vi "Data Access.vi"(8 "error in (no error)":errorcluster, 10 "Data Access Handler":refnum<class "Data Access Handler.lvclass">, 11 "List Instrument Msg in":refnum<class "List Instruments Msg.lvclass">) -> (0 "error out":errorcluster, 3 "List Instrument Msg out":refnum<class "List Instruments Msg.lvclass">)   [LabVIEW 2020, in "Instrument Handler.lvlib" / "List Instruments Msg.lvclass"]
doc: "Expose class private data to the front panel while letting the Data Access Handler class act on the data."
uses:
  List Instruments Msg.lvclass
  C:/Current projects/WS/Framework/Framework/Actors/Instrument Handler/Instrument Handler Messages/Instrument Handler Response Msg/Instrument Handler Response Msg.lvclass
  C:/Current projects/WS/PPL/HDH.Actor Framework.Core.Msg.lvlibp/Flex Msg/Flex Msg.lvclass
  PPL/HDH.Actor Framework.Core.Msg.lvlibp/Flex Msg/Data Access Handlers/Data Access Handler/Data Access Handler.lvclass
  PPL/HDH.Actor Framework.Core.Publisher.lvlibp/Messages/Response Msg/Response Core/Controls/Ctl_SendFunction.ctl
  PPL/HDH.Actor Framework.Core.Actor.lvlibp/1abvi3w/vi.lib/ActorFramework/Message Enqueuer/Message Priority.ctl
  Instrument Handler Response Msg/Instrument Handler Response Msg.lvclass/Instrument Handler Response Msg.ctl
  Instrument Handler Response Msg/Instrument Handler Response Msg.lvclass
  PPL/HDH.Actor Framework.Core.Publisher.lvlibp
  PPL/HDH.Actor Framework.Core.Actor.lvlibp/1abvi3w/vi.lib/ActorFramework/Message Enqueuer/Message Enqueuer.lvclass
panel:
  in  "Message Priority":T1=enum."Normal"
  in  "Send Function(Await Reply)":T2=enum."Await Reply"
  in  "Timeout if Waiting(-1ms)":i32=-1
  in  "Publish Data?(T)":bool=TRUE
  in  "Cancel":bool
  in  "OK":bool
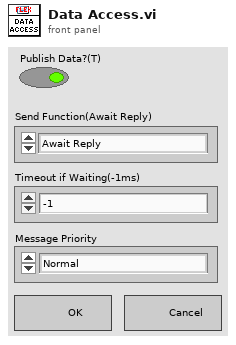
[diagram p1: front panel]
types:
  T1 = typedef "HDH.Actor Framework.Core.Actor.lvlibp/Message Enqueuer.lvclass/Message Priority.ctl" = enum16{"Low", "Normal", "High"}
  T2 = typedef "HDH.Actor Framework.Core.Publisher.lvlibp/Ctl_SendFunction.ctl" = enum16{"Send and Forget", "Request Reply", "Await Reply"}
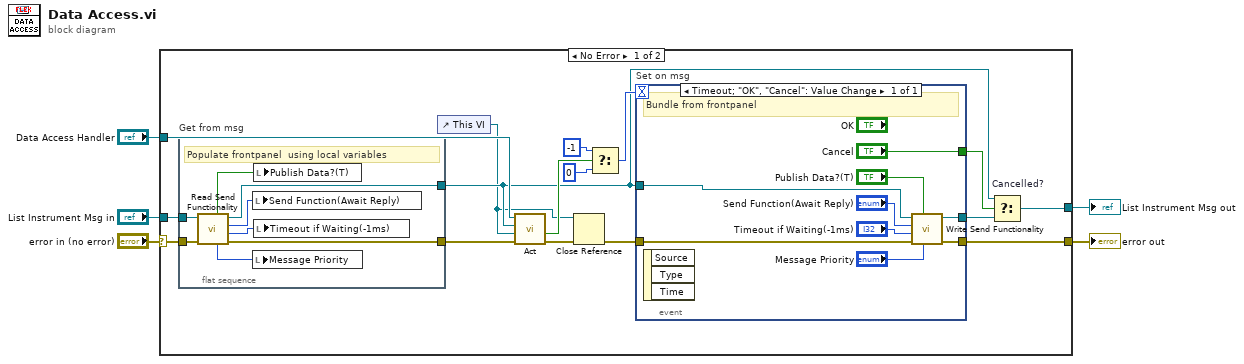
[diagram p0: block diagram]
diagram:
  n1 = case shown="No Error" "error in (no error)" {
    selector: "error in (no error)" -> [w21 w40]
    tunnel: [w14 w40] -> w4
    tunnel: [w9 w39] -> w2
    tunnel: "List Instrument Msg in" -> [w12 w39]
    tunnel: "Data Access Handler" -> [w20 _]
    frame No Error {
      n2 = flat-sequence "Get from msg" {
        tunnel: w21 -> [w38]
        tunnel: [w35] -> w7
        tunnel: w12 -> [w36]
        tunnel: [w37] -> w19
        frame #0 {
          # "Populate frontpanel  using local variables"
          n3 = call "Read Send Functionality.vi"("error in (no error)"=w38, "Instrument Handler Reponse Msg in"=w36) -> ("error out"=w37:errorcluster, "Timeout if Waiting"=w32:i32, "Send Function"=w33:T2, "Instrument Handler Reponse Msg out"=w35:refnum<class "List Instruments Msg.lvclass">, "Message Priority"=w31:T1, "Publish Data?"=w34:bool)  [unwired: 4 in]
          n4 = local write "Send Function(Await Reply)"(w33) -> ()
          n5 = local write "Message Priority"(w31) -> ()
          n6 = local write "Publish Data?(T)"(w34) -> ()
          n7 = local write "Timeout if Waiting(-1ms)"(w32) -> ()
        }
      }
      n8 = control-ref of="This VI"() -> (w6:refnum<vi>)
      n9 = call-dynamic "Act.vi"("error in (no error)"=w19, "VI Refnum in"=w6, "Flex Msg type"=w7, "Data Access Handler in"=w20) -> ("error out"=w11:errorcluster, "Await user action?"=w18:bool)  [unwired: 5 in, 1 out]
      n10 = Close Reference(reference=w6, error in (no error)=w11) -> (error out=w13:errorcluster)
      n11 = Select(t=-1, s=w18, f=0 ("t")) -> (s? t:f=w15:i32)
      n12 = event "Set on msg" shown="[0] Timeout;  \"OK\", \"Cancel\": Value Change" {
        selector: _ -> [_]
        dyn-events: _ -> [_]
        timeout: w15 -> [_]
        tunnel: [w28] -> w14
        tunnel: w13 -> [w30]
        tunnel: ["Cancel"] -> w10
        tunnel: [w26] -> w8
        tunnel: w7 -> [w27]
        event Timeout; "OK", "Cancel": Value Change {
          # "Bundle from frontpanel"
          n13 = event-data() -> ()  [unwired: 1 in, 3 out]
          n14 = call "Write Send Functionality.vi"("Message Priority"="Message Priority", "Publish Data?(T)"="Publish Data?(T)", "error in (no error)"=w30, "Timeout if Waiting(-1ms)"="Timeout if Waiting(-1ms)", "Send Function(Await Reply)"="Send Function(Await Reply)", "Instrument Handler Reponse Msg in"=w27) -> ("error out"=w28:errorcluster, "Instrument Handler Reponse Msg out"=w26:refnum<class "List Instruments Msg.lvclass">)  [unwired: 4 in]
        }
      }
      n15 = Select "Cancelled?"(t=w7, s=w10, f=w8) -> (s? t:f=w9:refnum<class "List Instruments Msg.lvclass">)
    }
    frame Error {
    }
  }
  "error out" <- w4
  "List Instrument Msg out" <- w2
